vi "下发产品测试信息给PLC.vi"(8 "错误in":errorcluster) -> (0 "错误out":errorcluster)   [LabVIEW 2014]
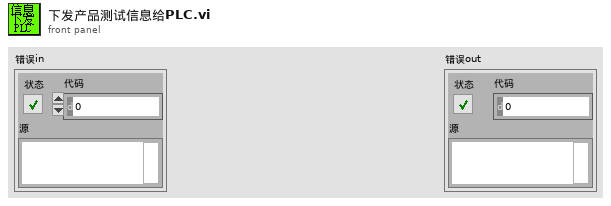
[diagram p1: front panel]
types:
  T1 = typedef "欧姆龙PLC Action.ctl" = enum16{"初始化", "重新初始化", "读触发信息", "读示教坐标P1P2", "读示教坐标P3P4", "读示教坐标P11P12", "读示教坐标P13P14", "读第1组Mark点坐标", "读第2组Mark点坐标", "读第3组Mark点坐标", "自检：写螺丝刀拍照结果和Finish", "自检：写供料盘二维码拍照结果和Finish", "读第4组Mark点坐标", "写取料点相对拍照点移动量", "写放料点坐标", "写放螺丝时相对当前拍照点偏移量", "写取料点相对拍照点移动量&放料点坐标", "写螺杆拍照完成Finish", "写读取锁附结果完成信号", "写复锁时相对拍照点移动量", "写数据-测试用", "写当前产品基本供料信息", "写当前产品每颗螺丝来自哪个供料盘", "写当前产品每颗螺丝拧紧程式序号", "写当前产品4个预锁程式和4个复锁程式序号", "写第1组Mark点坐标", "写第2组Mark点坐标", "写第3组Mark点坐标", "写第4组Mark点坐标", "写夹螺杆点到拍螺帽点距离", "写第1组复锁拍照点", "写第2组复锁拍照点", "写第3组复锁拍照点", "写第4组复锁拍照点", "写启用的托盘螺丝拧紧程式参数", "写预锁复锁拧紧程式参数", "获取信息"}
  T2 = typedef "欧姆龙PLC Action.ctl" = enum16{"读设备状态", "初始化", "待命", "重新初始化", "读触发信息", "读第1组Mark点坐标", "读第2组Mark点坐标", "写基本信息", "写第1组Mark点坐标", "写第2组Mark点坐标", "写相机中心到出线头的距离", "写一笔轨迹到PLC", "写入进线前段点位", "写入板内布线点位", "写入出线布线点位", "写入数据写入完成信号", "获取信息", "写入进出线方向", "写加工信号"}
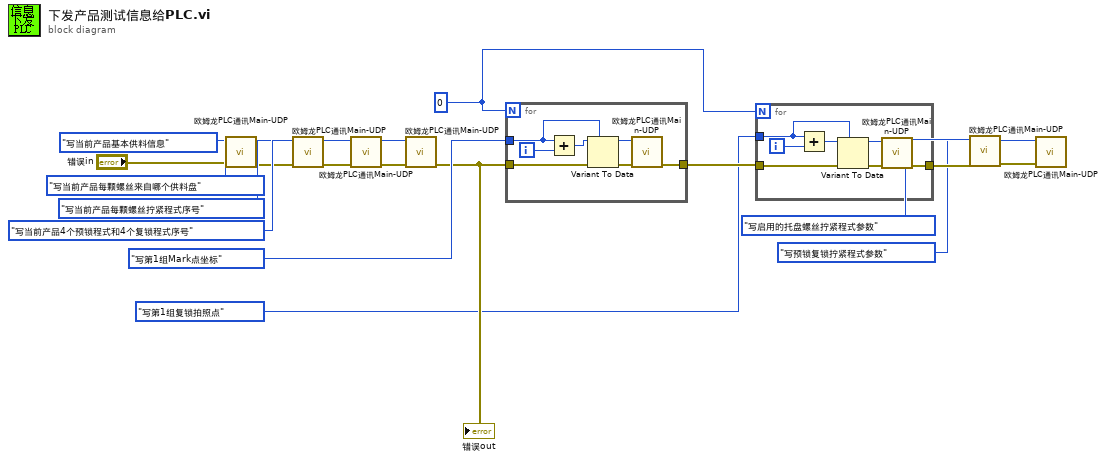
[diagram p0: block diagram]
diagram:
  w1 = 0
  n1 = call "欧姆龙PLC通讯Main-UDP.vi"("错误in"="错误in", "欧姆龙PLC Action"=欧姆龙PLC_Action."写当前产品基本供料信息") -> ("错误out"=w11:errorcluster)  [unwired: 7 in, 2 out]
  n2 = call "欧姆龙PLC通讯Main-UDP.vi"("错误in"=w11, "欧姆龙PLC Action"=欧姆龙PLC_Action."写当前产品每颗螺丝来自哪个供料盘") -> ("错误out"=w12:errorcluster)  [unwired: 7 in, 2 out]
  n3 = call "欧姆龙PLC通讯Main-UDP.vi"("错误in"=w12, "欧姆龙PLC Action"=欧姆龙PLC_Action."写当前产品每颗螺丝拧紧程式序号") -> ("错误out"=w13:errorcluster)  [unwired: 7 in, 2 out]
  n4 = call "欧姆龙PLC通讯Main-UDP.vi"("错误in"=w13, "欧姆龙PLC Action"=欧姆龙PLC_Action."写当前产品4个预锁程式和4个复锁程式序号") -> ("错误out"=w16:errorcluster)  [unwired: 7 in, 2 out]
  "错误out" <- w16
  n5 = for {
    N: w1 -> [_]
    tunnel: w16 -> [w21]
    tunnel: 欧姆龙PLC_Action."写第1组Mark点坐标" ("欧姆龙PLC Action") -> [w24]
    tunnel: [w18] -> w7
    i -> [w19]
    n6 = Add(x=w24, y=w19) -> (x+y=w23:i32)
    n7 = Variant To Data(error in=w21, type=w24, Variant=w23) -> (data=w22:T2, error out=w20:errorcluster)
    n8 = call "欧姆龙PLC通讯Main-UDP.vi"("错误in"=w20, "欧姆龙PLC Action"=w22) -> ("错误out"=w18:errorcluster)  [unwired: 7 in, 2 out]
  }
  n9 = for {
    N: w1 -> [_]
    tunnel: w7 -> [w28]
    tunnel: 欧姆龙PLC_Action."写第1组复锁拍照点" ("欧姆龙PLC Action") -> [w31]
    tunnel: [w25] -> w5
    i -> [w26]
    n10 = Add(x=w31, y=w26) -> (x+y=w30:i32)
    n11 = Variant To Data(error in=w28, type=w31, Variant=w30) -> (data=w29:T1, error out=w27:errorcluster)
    n12 = call "欧姆龙PLC通讯Main-UDP.vi"("错误in"=w27, "欧姆龙PLC Action"=w29) -> ("错误out"=w25:errorcluster)  [unwired: 7 in, 2 out]
  }
  n13 = call "欧姆龙PLC通讯Main-UDP.vi"("错误in"=w5, "欧姆龙PLC Action"=欧姆龙PLC_Action."写启用的托盘螺丝拧紧程式参数") -> ("错误out"=w3:errorcluster)  [unwired: 7 in, 2 out]
  n14 = call "欧姆龙PLC通讯Main-UDP.vi"("错误in"=w3, "欧姆龙PLC Action"=欧姆龙PLC_Action."写预锁复锁拧紧程式参数") -> ()  [unwired: 7 in, 3 out]
